vi "Initialize RT Driver.vi"(8 "error in":errorcluster, 10 "settings in":T18 {"objectData"."out object status BD"."Data Reference" format="%.0x"; "objectData"."out object data BD"."Data Reference" format="%.0x"; "objectData"."out interaction status BD"."Data Reference" format="%.0x"; "objectData"."out interaction data BD"."Data Reference" format="%.0x"}, 11 "Device Reference in":T25 format="%.0x") -> (0 "error out":errorcluster, 1 "inline runtime data":T1 {"out object status BD"."Data Reference" format="%.0x"; "out object data BD"."Data Reference" format="%.0x"; "out interaction status BD"."Data Reference" format="%.0x"; "out interaction data BD"."Data Reference" format="%.0x"}, 2 "settings out":T18 {"objectData"."out object status BD"."Data Reference" format="%.0x"; "objectData"."out object data BD"."Data Reference" format="%.0x"; "objectData"."out interaction status BD"."Data Reference" format="%.0x"; "objectData"."out interaction data BD"."Data Reference" format="%.0x"}, 3 "Device Reference out":T25 format="%.0x")   [LabVIEW 2019, in "HLA Custom Device Engine.lvlib"]
uses:
  HLA Custom Device Engine.lvlib
  <vilib>/NI VeriStand/Custom Device API/Custom Device Item Ref.ctl
  Shared/Compiled.Settings.ctl
  Shared/main_page_config.ctl
  Shared/object_managament_config.ctl
  Shared/interaction_parameter_configuration.ctl
  Shared/object_attribute_configuration.ctl
  Shared/object_status_info.ctl
  Shared/object_data.ctl
  <vilib>/NI VeriStand/Custom Device API/Block Data Reference.ctl
  <vilib>/NI VeriStand/Custom Device API/Data Reference.ctl
  RTruntimeData.ctl
  _typedefs/RThlaMapHelpers.ctl
  _typedefs/map_in_interaction.ctl
  _typedefs/map_interaction_value.ctl
  _typedefs/map_attr_param_data.ctl
  _typedefs/map_object.ctl
  _typedefs/map_object_key.ctl
  _typedefs/map_object_value.ctl
  _typedefs/map_object_instance.ctl
  _typedefs/map_object_instance_value.ctl
  _typedefs/map_object_vs_instance.ctl
  _typedefs/map_out_vs_ch_instanceId.ctl
  _typedefs/map_out_vs_ch_objects.ctl
  _typedefs/map_out_vs_ch_objects_value.ctl
  _typedefs/map_out_vs_ch_interactIonClass.ctl
  <vilib>/addons/hla/receiveInteractionEvent_type.ctl
  <vilib>/addons/hla/OrderType.ctl
  <vilib>/addons/hla/TransportationType.ctl
  <vilib>/addons/hla/reflectAttributeValuesEvent_type.ctl
  <vilib>/addons/hla/discoverObjectInstanceEvent_type.ctl
  <vilib>/addons/hla/removeObjectInstanceEvent_type.ctl
  Shared/rt_init_state.ctl
  <vilib>/Utility/miscctls.llb/LVMapReplaceAction.ctl
  _typedefs/discoverObjectInstance_type.ctl
  <vilib>/NI VeriStand/Custom Device API/Custom Device API.lvlib
  <vilib>/addons/hla/openrti_rti1516eLv.lvlib
  Shared/HLA Custom Device Shared.lvlib
  _Debug/VsDebugLibrary.lvlib
  <vilib>/addons/hla/helpers/ahs.lvlib
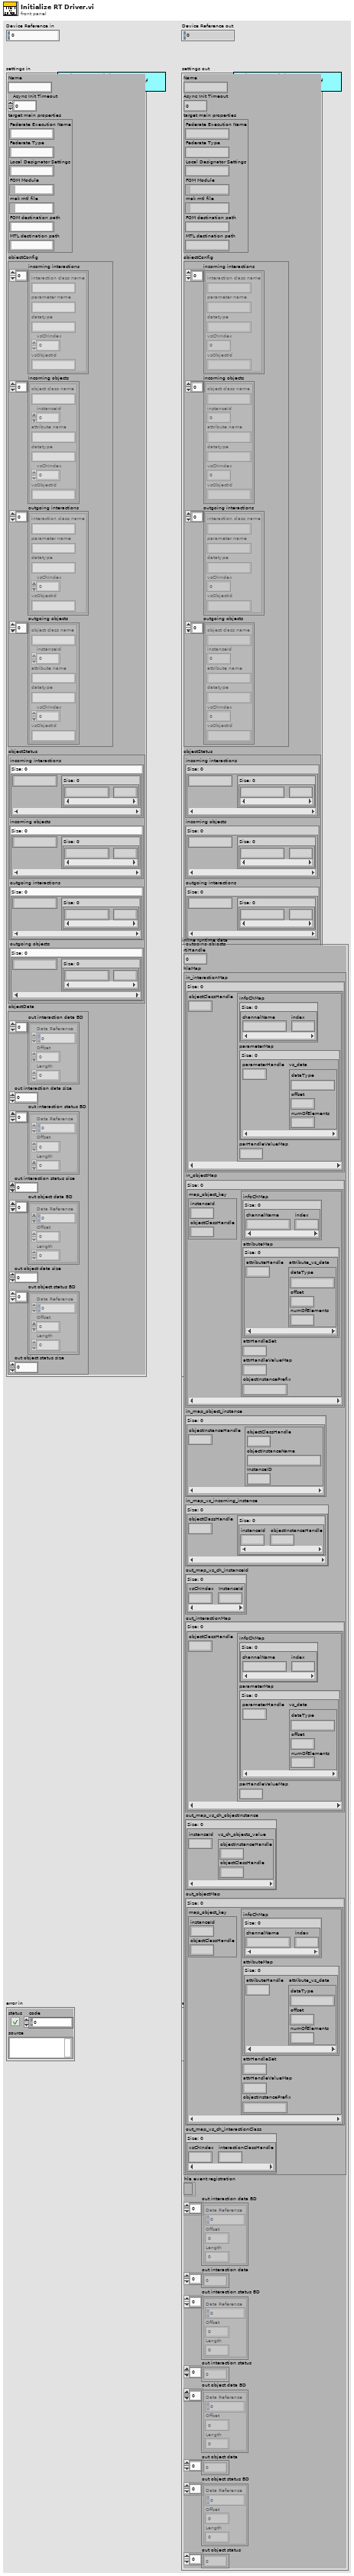
[diagram p1: front panel]
types:
  T1 = typedef "HLA Custom Device Engine.lvlib/RTruntimeData.ctl" = cluster{"rtiHandle":i64, "hlaMap":T2, "hla event registration":refnum<event-registration>, "out interaction data BD":T16[], "out interaction data":dbl[], "out interaction status BD":T16[], "out interaction status ":dbl[], "out object data BD":T16[], "out object data":dbl[], "out object status BD":T16[], "out object status ":dbl[]}
  T2 = typedef "HLA Custom Device Engine.lvlib/RThlaMapHelpers.ctl" = cluster{"in_interactionMap":T3, "in_objectMap":T6, "in_map_object_instance":T9, "in_map_vs_incoming_instance":T11, "out_map_vs_ch_instanceId":T12, "out_interactionMap":T3, "out_map_vs_ch_objectInstance":T13, "out_objectMap":T6, "out_map_vs_ch_interactionClass":T15}
  T3 = typedef "HLA Custom Device Engine.lvlib/map_in_interaction.ctl" = map{u64, T4}
  T4 = typedef "HLA Custom Device Engine.lvlib/map_interaction_value.ctl" = cluster{"infoChMap":map{string, i32}, "parameterMap":map{u64, T5}, "parHandleValueMap":u64}
  T5 = typedef "HLA Custom Device Engine.lvlib/map_attr_param_data.ctl" = cluster{"dataType":string, "offset":i32, "numOfElements":i32}
  T6 = typedef "HLA Custom Device Engine.lvlib/map_object.ctl" = map{T7, T8}
  T7 = typedef "HLA Custom Device Engine.lvlib/map_object_key.ctl" = cluster{"instanceId":i32, "objectClassHandle":u64}
  T8 = typedef "HLA Custom Device Engine.lvlib/map_object_value.ctl" = cluster{"infoChMap":map{string, i32}, "attributeMap":map{u64, T5}, "attrHandleSet":u64, "attrHandleValueMap":u64, "objectInstancePrefix":string}
  T9 = typedef "HLA Custom Device Engine.lvlib/map_object_instance.ctl" = map{u64, T10}
  T10 = typedef "HLA Custom Device Engine.lvlib/map_object_instance_value.ctl" = cluster{"objectClassHandle":u64, "objectInstanceName":string, "InstanceID":i32}
  T11 = typedef "HLA Custom Device Engine.lvlib/map_object_vs_instance.ctl" = map{u64, map{i32, u64}}
  T12 = typedef "HLA Custom Device Engine.lvlib/map_out_vs_ch_instanceId.ctl" = map{i32, i32}
  T13 = typedef "HLA Custom Device Engine.lvlib/map_out_vs_ch_objects.ctl" = map{i32, T14}
  T14 = typedef "HLA Custom Device Engine.lvlib/map_out_vs_ch_objects_value.ctl" = cluster{"objectInstanceHandle":u64, "objectClassHandle":u64}
  T15 = typedef "HLA Custom Device Engine.lvlib/map_out_vs_ch_interactIonClass.ctl" = map{i32, u64}
  T16 = typedef "Custom Device API.lvlib/Block Data Reference.ctl" = cluster{"Data Reference":T17, "Offset":u64, "Length":u64}
  T17 = typedef "Custom Device API.lvlib/Data Reference.ctl" = i32
  T18 = typedef "HLA Custom Device Shared.lvlib/Compiled.Settings.ctl" = cluster{"Name":string, "Async Init Timeout":u16, "target main properties":T19, "obiectConfig":T20, "objectStatus":T23, "objectData":T24}
  T19 = typedef "HLA Custom Device Shared.lvlib/main_page_config.ctl" = cluster{"Federate Execution Name":string, "Federate Type":string, "Local Designator Settings":string, "FOM Module":path, "mak mtl file":path, "FOM destination path":string, "MTL destination path":string}
  T20 = typedef "HLA Custom Device Shared.lvlib/object_managament_config.ctl" = cluster{"incoming interactions":T21[], "incoming objects":T22[], "outgoing interactions":T21[], "outgoing objects":T22[]}
  T21 = typedef "HLA Custom Device Shared.lvlib/interaction_parameter_configuration.ctl" = cluster{"interaction class name":string, "parameter name":string, "datatype":string, "vsChIndex":i32, "vsObjectId":string}
  T22 = typedef "HLA Custom Device Shared.lvlib/object_attribute_configuration.ctl" = cluster{"object class name":string, "instanceId":i32, "attribute name":string, "datatype":string, "vsChIndex":i32, "vsObjectId":string}
  T23 = typedef "HLA Custom Device Shared.lvlib/object_status_info.ctl" = cluster{"incoming interactions":map{string, map{string, i32}}, "incoming objects":map{string, map{string, i32}}, "outgoing interactions":map{string, map{string, i32}}, "outgoing objects":map{string, map{string, i32}}}
  T24 = typedef "HLA Custom Device Shared.lvlib/object_data.ctl" = cluster{"out interaction data BD":T16[], "out interaction data size":i32, "out interaction status BD":T16[], "out interaction status size":i32, "out object data BD":T16[], "out object data size":i32, "out object status BD":T16[], "out object status size":i32}
  T25 = typedef "Custom Device API.lvlib/Custom Device Item Ref.ctl" = u64
  T26 = typedef "HLA Custom Device Shared.lvlib/rt_init_state.ctl" = enum16{"Initialize", "Connect", "FOM Management", "Object Management", "Start", "RegisterObjectInstances"}
  T27 = cluster{"objInstanceName":string, "success":bool}
  T28 = typedef "LVMapReplaceAction.ctl" = enum32{"Modify Entry only if found", "Add or Modify Entry", "Delete Entry"}
  T29 = typedef "HLA Custom Device Engine.lvlib/discoverObjectInstance_type.ctl" = cluster{"objectInstanceHandle":u64, "objectClassHandle":u64, "objectInstanceName":string}
  T30 = cluster{"[0]":u8, "[1]":u8, "[2]":u8, "[3]":u8, "[4]":u8, "[5]":u8, "[6]":u8, "[7]":u8, "[8]":u8, "[9]":u8, "[10]":u8, "[11]":u8, "[12]":u8, "[13]":u8, "[14]":u8, "[15]":u8, "[16]":u8, "[17]":u8, "[18]":u8, "[19]":u8, "[20]":u8, "[21]":u8, "[22]":u8, "[23]":u8, "[24]":u8, "[25]":u8, "[26]":u8, "[27]":u8, "[28]":u8, "[29]":u8, "[30]":u8, "[31]":u8, "[32]":u8, "[33]":u8, "[34]":u8, "[35]":u8, "[36]":u8, "[37]":u8, "[38]":u8, "[39]":u8, "[40]":u8, "[41]":u8, "[42]":u8, "[43]":u8, "[44]":u8, "[45]":u8, "[46]":u8, "[47]":u8, "[48]":u8, "[49]":u8, "[50]":u8, "[51]":u8, "[52]":u8, "[53]":u8, "[54]":u8, "[55]":u8, "[56]":u8, "[57]":u8, "[58]":u8, "[59]":u8, "[60]":u8, "[61]":u8, "[62]":u8, "[63]":u8, "[64]":u8, "[65]":u8, "[66]":u8, "[67]":u8, "[68]":u8, "[69]":u8, "[70]":u8, "[71]":u8, "[72]":u8, "[73]":u8, "[74]":u8, "[75]":u8, "[76]":u8, "[77]":u8, "[78]":u8, "[79]":u8, "[80]":u8, "[81]":u8, "[82]":u8, "[83]":u8, "[84]":u8, "[85]":u8, "[86]":u8, "[87]":u8, "[88]":u8, "[89]":u8, "[90]":u8, "[91]":u8, "[92]":u8, "[93]":u8, "[94]":u8, "[95]":u8, "[96]":u8, "[97]":u8, "[98]":u8, "[99]":u8, "[100]":u8, "[101]":u8, "[102]":u8, "[103]":u8, "[104]":u8, "[105]":u8, "[106]":u8, "[107]":u8, "[108]":u8, "[109]":u8, "[110]":u8, "[111]":u8, "[112]":u8, "[113]":u8, "[114]":u8, "[115]":u8, "[116]":u8, "[117]":u8, "[118]":u8, "[119]":u8, "[120]":u8, "[121]":u8, "[122]":u8, "[123]":u8, "[124]":u8, "[125]":u8, "[126]":u8, "[127]":u8}
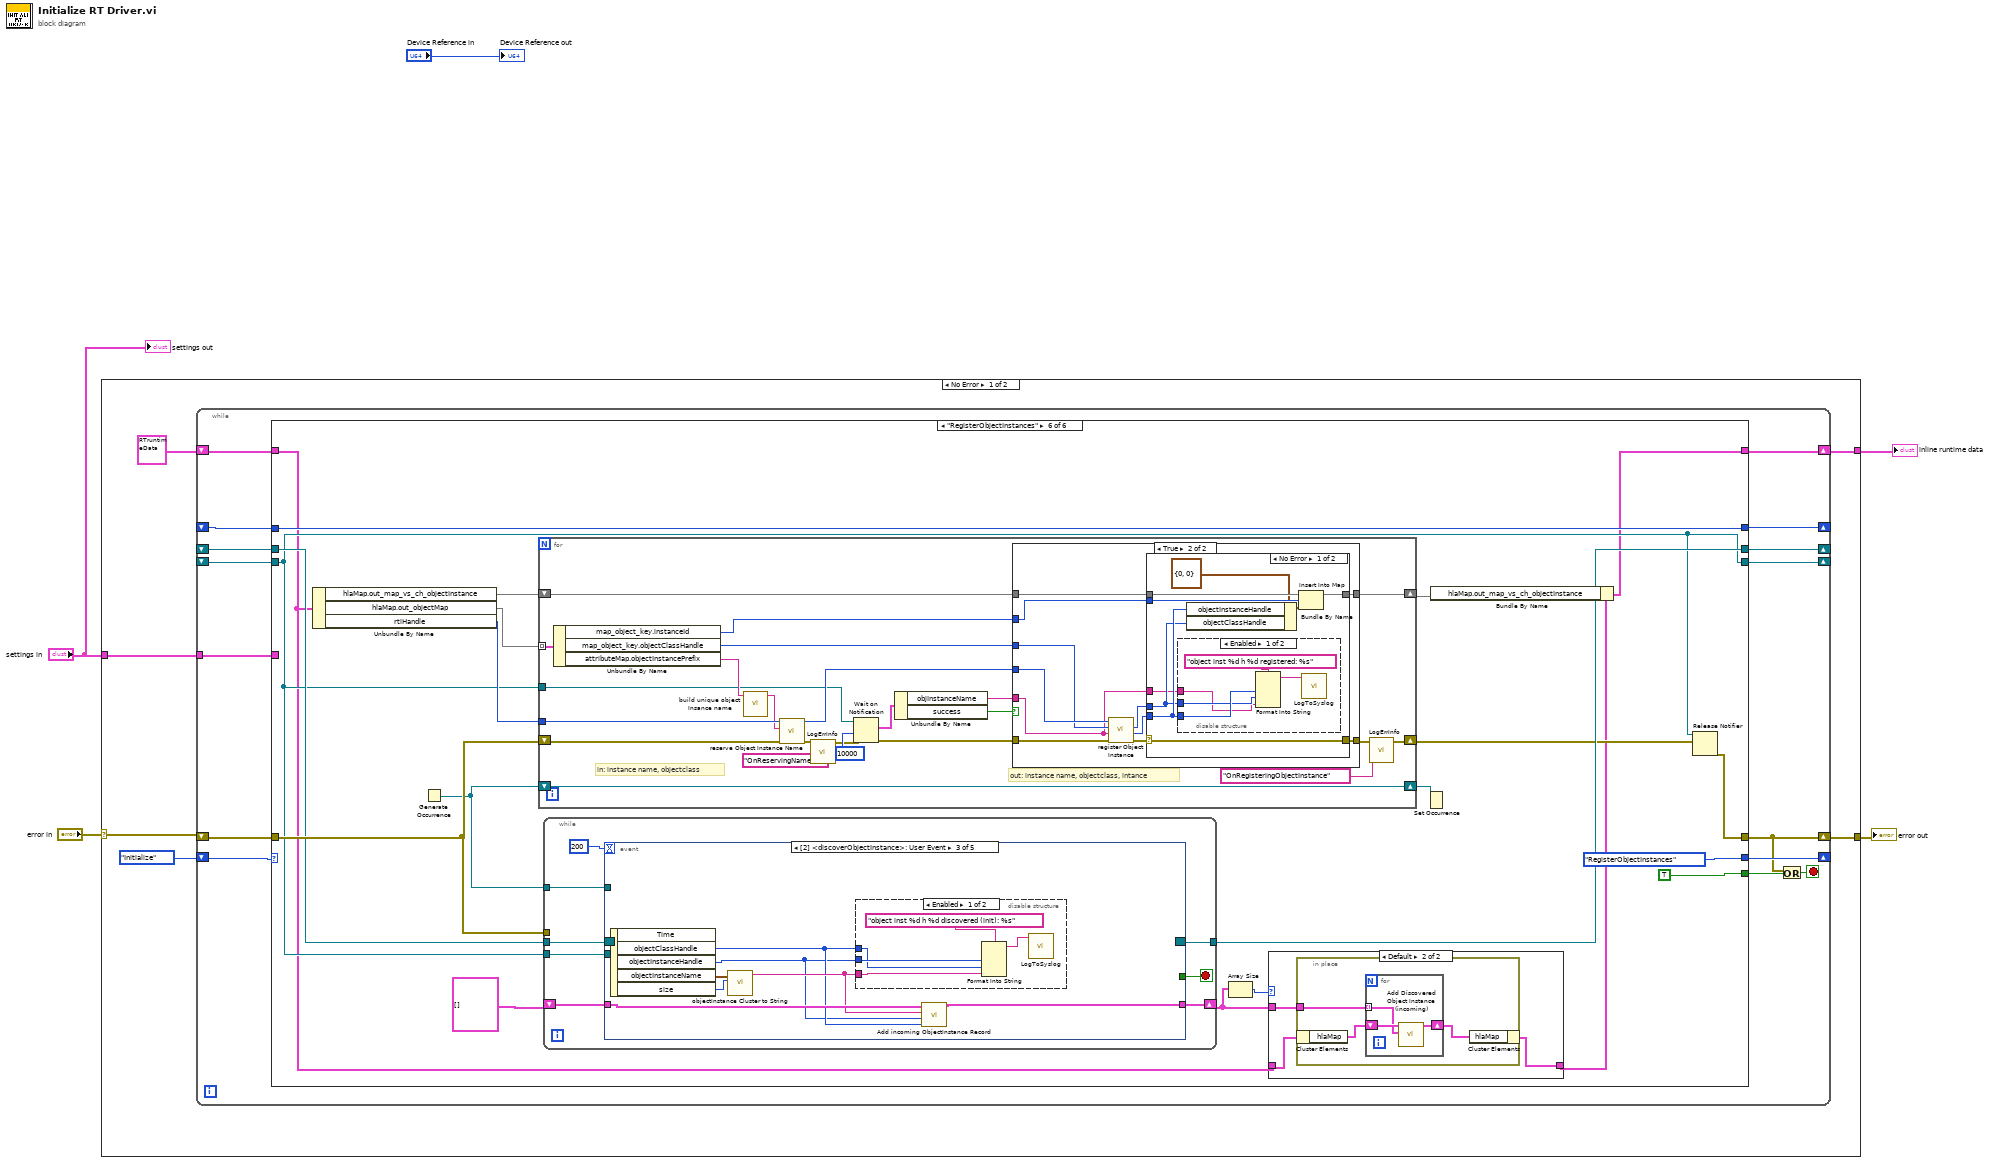
[diagram p0: block diagram]
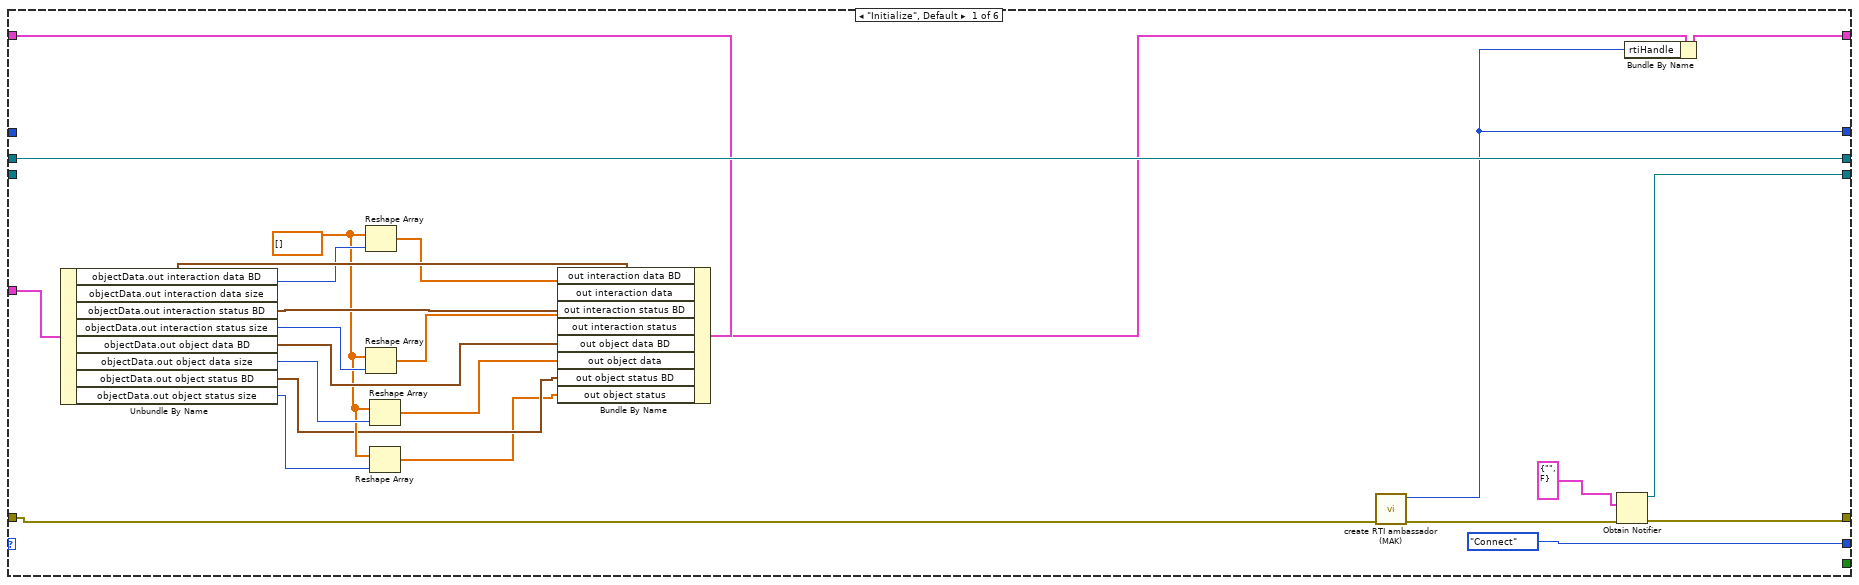
[diagram p2: hidden frame]
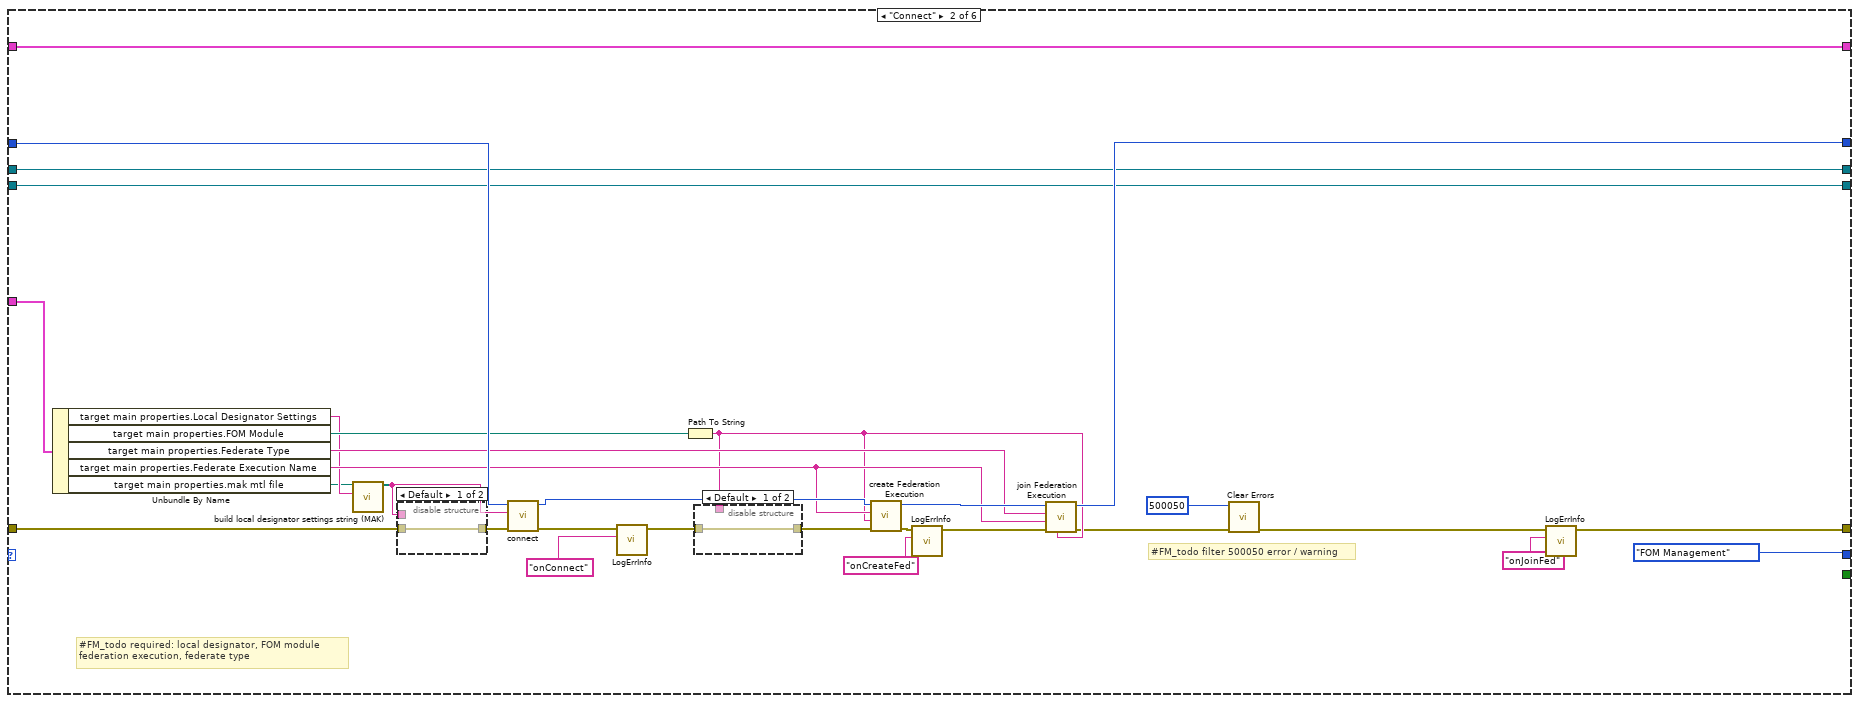
[diagram p3: hidden frame]
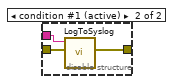
[diagram p4: hidden frame]
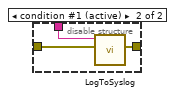
[diagram p5: hidden frame]
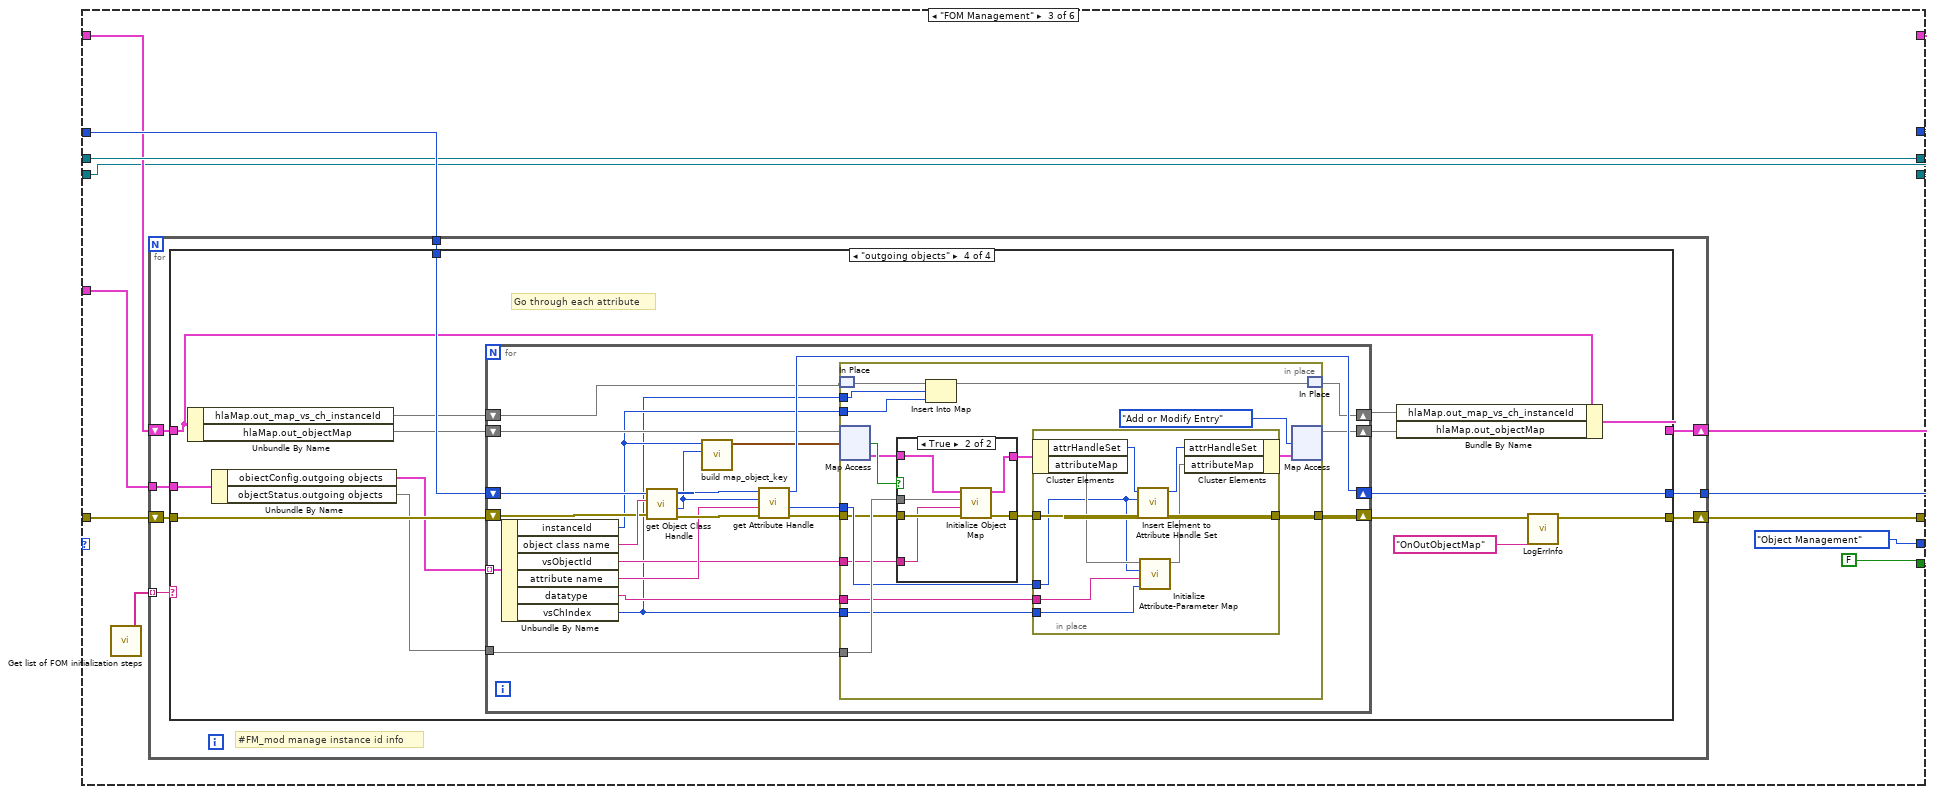
[diagram p6: hidden frame]
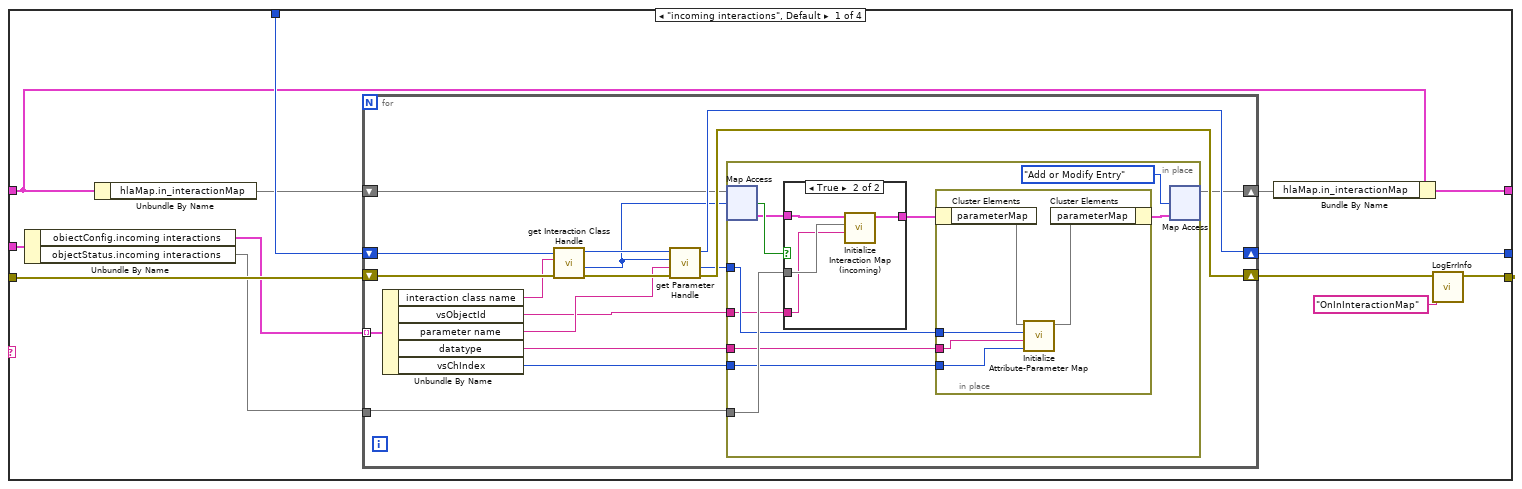
[diagram p7: hidden frame]
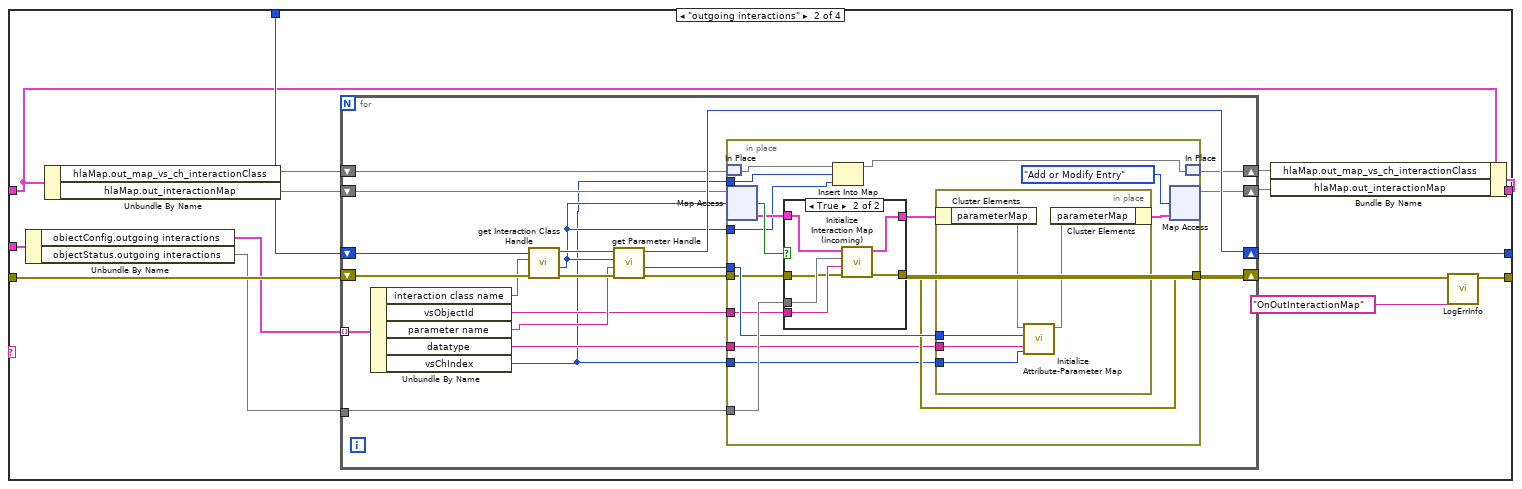
[diagram p9: hidden frame]
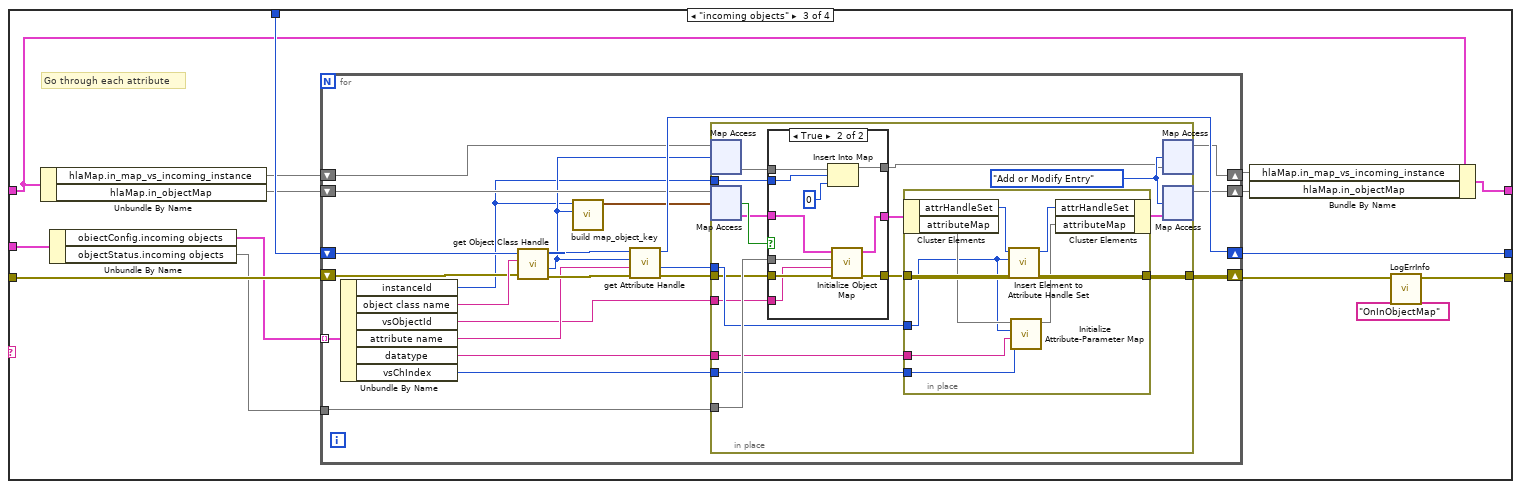
[diagram p11: hidden frame]
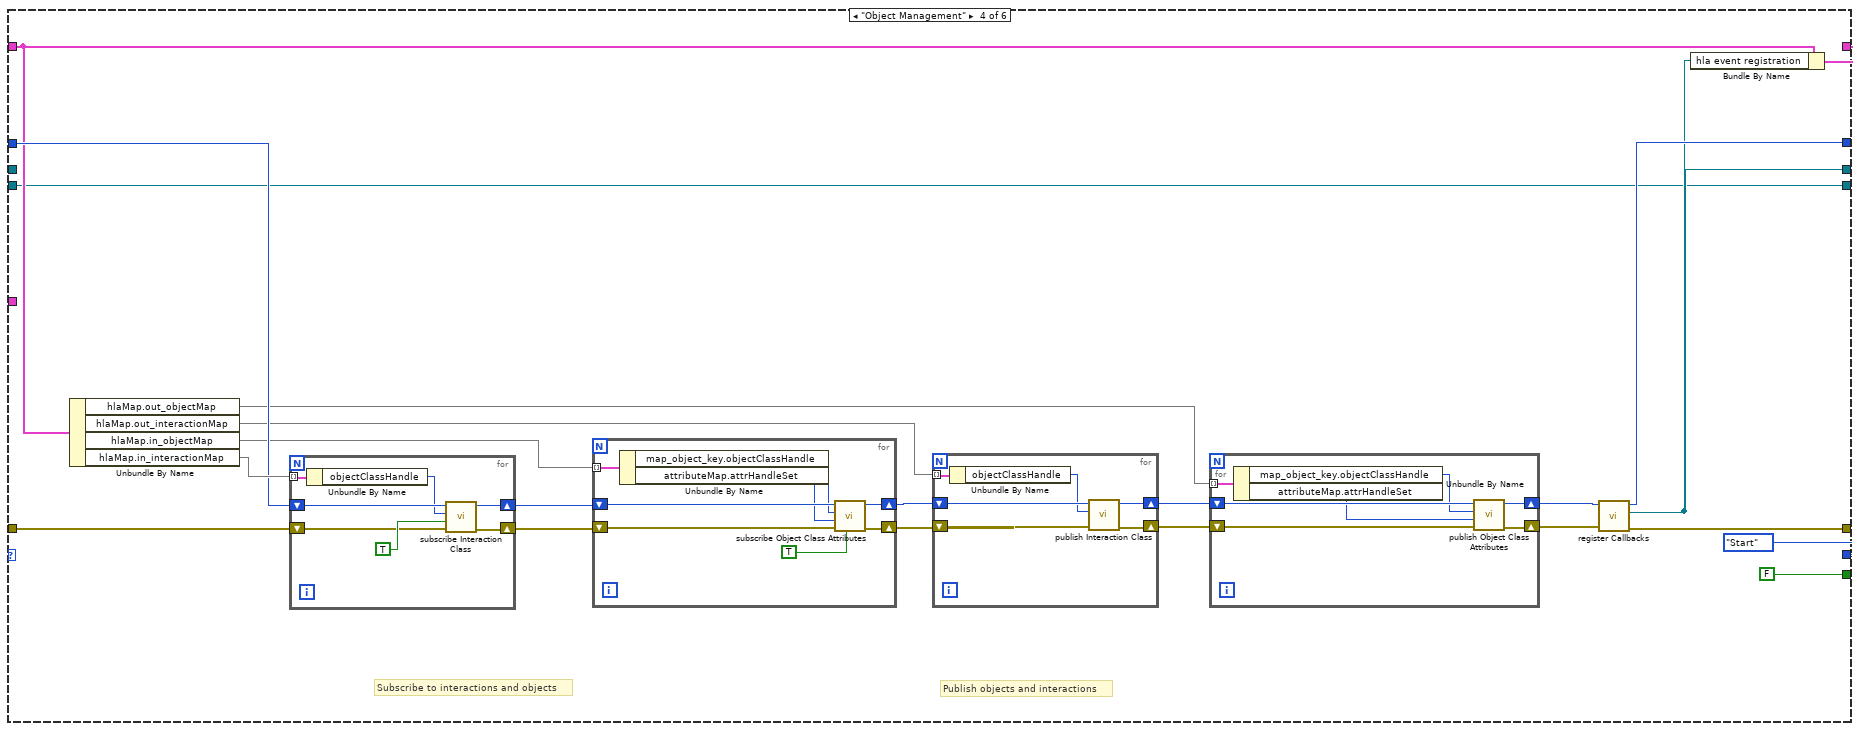
[diagram p14: hidden frame]
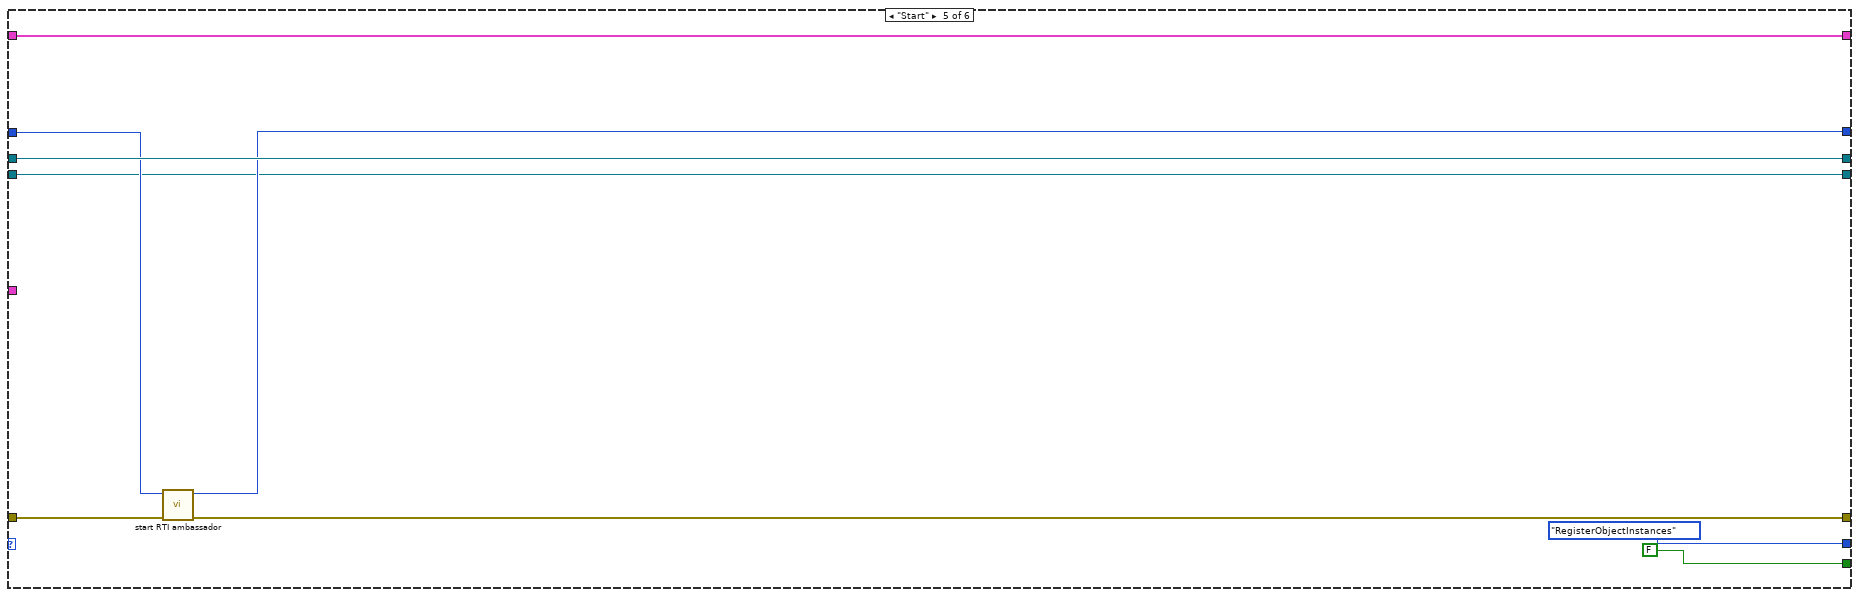
[diagram p15: hidden frame]
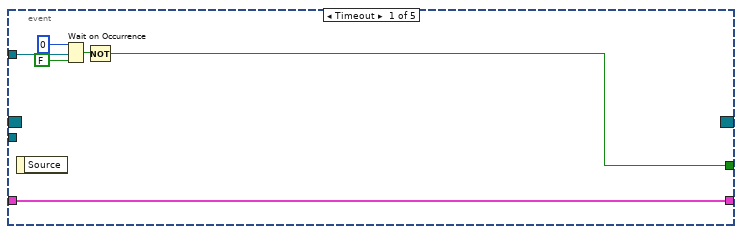
[diagram p20: hidden frame]
diagram:
  n1 = case shown="No Error" "error in" {
    selector: "error in" -> [w10 w559]
    tunnel: "settings in" -> [w9 _]
    tunnel: [w8 w559] -> w2
    tunnel: [w6 _] -> w1
    frame No Error {
      n2 = while {
        shift-right: [w25] -> _
        shift-left: rt_init_state."Initialize" -> [w26]
        tunnel: w9 -> [w24]
        shift-right: [w19] -> w8
        shift-left: w10 -> [w23]
        shift-right: [w22] -> _
        shift-left: _ -> [w21]
        shift-right: [w17] -> _
        shift-left: _ -> [w16]
        shift-right: [w14] -> w6
        shift-left: T1 {"rtiHandle"=0, "hlaMap"={"in_interactionMap"={}, "in_objectMap"={}, "in_map_object_instance"={}, "in_map_vs_incoming_instance"={}, "out_map_vs_ch_instanceId"={}, "out_interactionMap"={}, "out_map_vs_ch_objectInstance"={}, "out_objectMap"={}, "out_map_vs_ch_interactionClass"={}}, "hla event registration"=refnum, "out interaction data BD"=[], "out interaction data"=[], "out interaction status BD"=[], "out interaction status "=[], "out object data BD"=[], "out object data"=[], "out object status BD"=[], "out object status "=[]} ("inline runtime data") -> [w15]
        shift-right: [w13] -> _
        shift-left: _ -> [w12]
        stop <- w18 stop-if-true
        n3 = case shown="\"RegisterObjectInstances\"" w26 {
          tunnel: [w36 w72 w96 w383 w423 w440] -> w19
          tunnel: [_ _ FALSE FALSE FALSE TRUE] -> w20
          tunnel: [rt_init_state."Connect" rt_init_state."FOM Management" rt_init_state."Object Management" rt_init_state."Start" rt_init_state."RegisterObjectInstances" rt_init_state."RegisterObjectInstances"] -> w25
          tunnel: w24 -> [w48 w56 w94 _ _ _]
          tunnel: w23 -> [w50 w63 w99 w389 w427 w445]
          tunnel: [w42 w75 w97 w386 w425 w449] -> w22
          tunnel: w21 -> [_ w80 w98 w387 w426 w449]
          tunnel: [w49 w55 w93 w380 w428 w446] -> w17
          tunnel: w16 -> [w49 w55 w93 _ w428 w443]
          tunnel: w15 -> [w47 w54 w92 w379 w421 w432]
          tunnel: [w43 w54 w91 w381 w421 w437] -> w14
          tunnel: [w35 w53 w90 w375 w420 w439] -> w13
          tunnel: w12 -> [_ w53 w90 w375 w420 w439]
          frame "Initialize", Default {
            w31 = dbl[] [] ("out interaction data")
            n4 = Unbundle By Name(w48) -> ("objectData.out interaction data BD"=w46:T16[], "objectData.out interaction data size"=w41:i32, "objectData.out interaction status BD"=w45:T16[], "objectData.out interaction status size"=w39:i32, "objectData.out object data BD"=w33:T16[], "objectData.out object data size"=w32:i32, "objectData.out object status BD"=w29:T16[], "objectData.out object status size"=w28:i32)
            n5 = Reshape Array(w31, w41) -> (w40:dbl[])
            n6 = Reshape Array(w31, w39) -> (w38:dbl[])
            n7 = Reshape Array(w31, w32) -> (w30:dbl[])
            n8 = Reshape Array(w31, w28) -> (w27:dbl[])
            n9 = Bundle By Name(cluster=w47, "out interaction data BD"=w46, "out interaction data"=w40, "out interaction status BD"=w45, "out interaction status"=w38, "out object data BD"=w33, "out object data"=w30, "out object status BD"=w29, "out object status"=w27) -> (w44:T1)
            n10 = call <vilib>:"create RTI ambassador (MAK).vi"("error in"=w50) -> ("error out"=w37:errorcluster, "rtiHandle out"=w42:i64)  [unwired: 9 in]
            n11 = Obtain Notifier(notification data type=T27 {"objInstanceName"="", "success"=FALSE} ("notification"), error in (no error)=w37) -> (notifier out=w35:refnum<notifier>, error out=w36:errorcluster)  [unwired: 2 in, 1 out]
            n12 = Bundle By Name(cluster=w44, "rtiHandle"=w42) -> (w43:T1)
          }
          frame "Connect" {
            # "#FM_todo filter 500050 error / warning"
            # "#FM_todo required: local designator, FOM module\nfederation execution, federate type"
            n13 = Unbundle By Name(w56) -> ("target main properties.Local Designator Settings"=w66:string, "target main properties.FOM Module"=w69:path, "target main properties.Federate Type"=w68:string, "target main properties.Federate Execution Name"=w67:string, "target main properties.mak mtl file"=w65:path)
            n14 = call "build local designator settings string (MAK).vi"("configuration string"=w66, "configuration file"=w65) -> ("local designator settings"=w64:string)  [unwired: 9 in]
            n15 = disable-structure shown="Default" {
              disable-tunnel: w64 -> [_ w85]
              disable-tunnel: w63 -> [w82 w84]
              disable-tunnel: [w82 w83] -> w62
              frame condition #0 {
              }
              frame condition #1 (active) {
                n16 = call "LogToSyslog.vi"("error in (no error)"=w84, "message"=w85) -> ("error out"=w83:errorcluster)  [unwired: 8 in, 1 out]
              }
            }
            n17 = call <vilib>:"connect.vi"("error in"=w62, "rtinode address"=w64, "rtiHandle in"=w80) -> ("error out"=w77:errorcluster, "rtiHandle out"=w76:i64)  [unwired: 7 in]
            n18 = call "LogErrInfo.vi"("location info"="onConnect", "error in (no error)"=w77) -> ("error out"=w61:errorcluster)  [unwired: 9 in]
            n19 = Path To String(path=w69) -> (string=w59:string)
            n20 = disable-structure shown="Default" {
              disable-tunnel: w61 -> [w86 w89]
              disable-tunnel: [w86 w88] -> w60
              disable-tunnel: w59 -> [_ w87]
              frame condition #0 {
              }
              frame condition #1 (active) {
                n21 = call "LogToSyslog.vi"("error in (no error)"=w89, "message"=w87) -> ("error out"=w88:errorcluster)  [unwired: 8 in, 1 out]
              }
            }
            n22 = call <vilib>:"create Federation Execution.vi"("error in"=w60, "fomModules"=w59, "federationExecutionName"=w67, "rtiHandle in"=w76) -> ("error out"=w78:errorcluster, "rtiHandle out"=w79:i64)  [unwired: 6 in]
            n23 = call "LogErrInfo.vi"("location info"="onCreateFed", "error in (no error)"=w78) -> ("error out"=w73:errorcluster)  [unwired: 9 in]
            n24 = call <vilib>:"join Federation Execution.vi"("additionalFomModules(\"\")"=w59, "error in"=w73, "federationExecutionName"=w67, "federateType"=w68, "rtiHandle in"=w79) -> ("error out"=w58:errorcluster, "rtiHandle out"=w75:i64)  [unwired: 5 in]
            n25 = call <vilib>:"Clear Errors.vi"("error in (no error)"=w58, "specific error code to clear (0: all)"=500050) -> ("error out"=w57:errorcluster)  [unwired: 4 in, 1 out]
            n26 = call "LogErrInfo.vi"("location info"="onJoinFed", "error in (no error)"=w57) -> ("error out"=w72:errorcluster)  [unwired: 9 in]
          }
          frame "FOM Management" {
            n27 = call "Get list of FOM initialization steps.vi"() -> ("init steps"=w95:string[])  [unwired: 11 in]
            n28 = for {
              tunnel: w94 -> [w109]
              tunnel: w98 -> [w107]
              tunnel: [w105] -> w97
              shift-right: [w103] -> w96
              shift-left: w99 -> [w108]
              shift-right: [w104] -> w91
              shift-left: w92 -> [w106]
              tunnel: w95 -> [w102] mode=indexing
              # "#FM_mod manage instance id info"
              n29 = case shown="\"outgoing objects\"" w102 {
                tunnel: w109 -> [w122 w174 w238 w313]
                tunnel: w108 -> [w121 w173 w237 w312]
                tunnel: w107 -> [w119 w171 w235 w310]
                tunnel: w106 -> [w117 w169 w233 w308]
                tunnel: [w116 w168 w232 w307] -> w105
                tunnel: [w115 w167 w231 w306] -> w104
                tunnel: [w112 w165 w228 w303] -> w103
                frame "incoming interactions", Default {
                  n30 = Unbundle By Name(w122) -> ("obiectConfig.incoming interactions"=w120:T21[], "objectStatus.incoming interactions"=w110:map{string, map{string, i32}})
                  n31 = Unbundle By Name(w117) -> ("hlaMap.in_interactionMap"=w118:T3)
                  n32 = for {
                    tunnel: w120 -> [w139] mode=indexing
                    shift-right: [w133] -> w116
                    shift-left: w119 -> [w137]
                    shift-right: [w132] -> w113
                    shift-left: w121 -> [w136]
                    shift-right: [w128] -> w114
                    shift-left: w118 -> [w131]
                    tunnel: w110 -> [w129]
                    n33 = Unbundle By Name(w139) -> ("interaction class name"=w126:string, "vsObjectId"=w125:string, "parameter name"=w134:string, "datatype"=w124:string, "vsChIndex"=w123:i32)
                    n34 = call <vilib>:"get Interaction Class Handle.vi"("error in"=w136, "interaction class name"=w126, "rtiHandle in"=w137) -> ("error out"=w138:errorcluster, "intClassHandle"=w130:u64, "rtiHandle out"=w135:i64)  [unwired: 6 in]
                    n35 = call <vilib>:"get Parameter Handle.vi"("error in"=w138, "theName"=w134, "intClassHandle"=w130, "rtiHandle in"=w135) -> ("error out"=w132:errorcluster, "parameterHandle"=w127:u64, "rtiHandle out"=w133:i64)  [unwired: 5 in]
                    n36 = in-place {
                      in-place-border: w129 -> [w148]
                      in-place-border: w127 -> [w144]
                      in-place-border: w125 -> [w142]
                      in-place-border: w124 -> [w141]
                      in-place-border: w123 -> [w140]
                      n37 = in-place-map #1(w131, w130) -> (w147:T4, w149:bool)  [unwired: 1 in]
                      n38 = case shown="True" w149 {
                        tunnel: w148 -> [_ w159]
                        tunnel: w147 -> [w155 w158]
                        tunnel: [w155 w157] -> w145
                        tunnel: w142 -> [_ w156]
                        frame False {
                        }
                        frame True {
                          n39 = call "Initialize Interaction Map (incoming).vi"("vsObjectId"=w156, "incoming interactions"=w159, "in_interaction map in"=w158) -> ("in_interaction map out"=w157:T4)  [unwired: 7 in, 1 out]
                        }
                      }
                      n40 = in-place {
                        in-place-border: w144 -> [w153]
                        in-place-border: w141 -> [w151]
                        in-place-border: w140 -> [w150]
                        n41 = in-place-cluster #2(w145) -> ("parameterMap"=w154:map{u64, T5})
                        n42 = call "Initialize Attribute-Parameter Map.vi"("vs channel index"=w150, "dataType"=w151, "parameterHandle"=w153, "Map in"=w154) -> ("Map out"=w152:map{u64, T5})  [unwired: 7 in]
                        n43 = in-place-cluster #2("parameterMap"=w152) -> (w143:T4)
                      }
                      n44 = in-place-map #1(w143, LVMapReplaceAction."Add or Modify Entry" ("action")) -> (w128:T3)  [unwired: 2 out]
                    }
                  }
                  n45 = Bundle By Name(cluster=w117, "hlaMap.in_interactionMap"=w114) -> (w115:T1)
                  n46 = call "LogErrInfo.vi"("location info"="OnInInteractionMap", "error in (no error)"=w113) -> ("error out"=w112:errorcluster)  [unwired: 9 in]
                }
                frame "outgoing interactions" {
                  n47 = Unbundle By Name(w174) -> ("obiectConfig.outgoing interactions"=w172:T21[], "objectStatus.outgoing interactions"=w163:map{string, map{string, i32}})
                  n48 = Unbundle By Name(w169) -> ("hlaMap.out_map_vs_ch_interactionClass"=w162:T15, "hlaMap.out_interactionMap"=w170:T3)
                  n49 = for {
                    tunnel: w172 -> [w194] mode=indexing
                    shift-right: [w188] -> w168
                    shift-left: w171 -> [w192]
                    shift-right: [w177] -> w166
                    shift-left: w173 -> [w191]
                    shift-right: [w185] -> w161
                    shift-left: w170 -> [w187]
                    tunnel: w163 -> [w186]
                    shift-right: [w179] -> w160
                    shift-left: w162 -> [w181]
                    n50 = Unbundle By Name(w194) -> ("interaction class name"=w183:string, "vsObjectId"=w182:string, "parameter name"=w189:string, "datatype"=w176:string, "vsChIndex"=w175:i32)
                    n51 = call <vilib>:"get Interaction Class Handle.vi"("error in"=w191, "interaction class name"=w183, "rtiHandle in"=w192) -> ("error out"=w193:errorcluster, "intClassHandle"=w180:u64, "rtiHandle out"=w190:i64)  [unwired: 6 in]
                    n52 = call <vilib>:"get Parameter Handle.vi"("error in"=w193, "theName"=w189, "intClassHandle"=w180, "rtiHandle in"=w190) -> ("error out"=w178:errorcluster, "parameterHandle"=w184:u64, "rtiHandle out"=w188:i64)  [unwired: 5 in]
                    n53 = in-place {
                      in-place-border: w186 -> [w209]
                      in-place-border: w184 -> [w205]
                      in-place-border: w182 -> [w203]
                      in-place-border: w175 -> [w198]
                      in-place-border: w180 -> [w197]
                      in-place-border: w178 -> [w202]
                      in-place-border: [w201] -> w177
                      in-place-border: w176 -> [w196]
                      in-place-border: w175 -> [w195]
                      n54 = in-place-match #3(w181) -> (w200:T15)
                      n55 = in-place-map #4(w187, w180) -> (w208:T4, w210:bool)  [unwired: 1 in]
                      n56 = case shown="True" w210 {
                        tunnel: w209 -> [_ w223]
                        tunnel: w208 -> [w217 w222]
                        tunnel: [w217 w221] -> w206
                        tunnel: w203 -> [_ w220]
                        tunnel: w202 -> [w216 w219]
                        tunnel: [w216 w218] -> w201
                        frame False {
                        }
                        frame True {
                          n57 = call "Initialize Interaction Map (incoming).vi"("error in"=w219, "vsObjectId"=w220, "incoming interactions"=w223, "in_interaction map in"=w222) -> ("error out"=w218:errorcluster, "in_interaction map out"=w221:T4)  [unwired: 6 in]
                        }
                      }
                      n58 = Insert Into Map(map in=w200, key=w198, value=w197) -> (map out=w199:T15)  [unwired: 2 out]
                      n59 = in-place {
                        in-place-border: w205 -> [w213]
                        in-place-border: w196 -> [w212]
                        in-place-border: w195 -> [w211]
                        n60 = in-place-cluster #5(w206) -> ("parameterMap"=w215:map{u64, T5})
                        n61 = call "Initialize Attribute-Parameter Map.vi"("vs channel index"=w211, "dataType"=w212, "parameterHandle"=w213, "Map in"=w215) -> ("Map out"=w214:map{u64, T5})  [unwired: 7 in]
                        n62 = in-place-cluster #5("parameterMap"=w214) -> (w204:T4)
                      }
                      n63 = in-place-map #4(w204, LVMapReplaceAction."Add or Modify Entry" ("action")) -> (w185:T3)  [unwired: 2 out]
                      n64 = in-place-match #3(w199) -> (w179:T15)
                    }
                  }
                  n65 = Bundle By Name(cluster=w169, "hlaMap.out_map_vs_ch_interactionClass"=w160, "hlaMap.out_interactionMap"=w161) -> (w167:T1)
                  n66 = call "LogErrInfo.vi"("location info"="OnOutInteractionMap", "error in (no error)"=w166) -> ("error out"=w165:errorcluster)  [unwired: 9 in]
                }
                frame "incoming objects" {
                  # "Go through each attribute"
                  n67 = Unbundle By Name(w233) -> ("hlaMap.in_map_vs_incoming_instance"=w225:T11, "hlaMap.in_objectMap"=w234:T6)
                  n68 = Unbundle By Name(w238) -> ("obiectConfig.incoming objects"=w236:T22[], "objectStatus.incoming objects"=w226:map{string, map{string, i32}})
                  n69 = for {
                    tunnel: w236 -> [w260] mode=indexing
                    shift-right: [w255] -> w232
                    shift-left: w235 -> [w258]
                    shift-right: [w247] -> w229
                    shift-left: w237 -> [w249]
                    shift-right: [w252] -> w230
                    shift-left: w234 -> [w254]
                    tunnel: w226 -> [w253]
                    shift-right: [w243] -> w224
                    shift-left: w225 -> [w245]
                    n70 = Unbundle By Name(w260) -> ("instanceId"=w242:i32, "object class name"=w250:string, "vsObjectId"=w239:string, "attribute name"=w256:string, "datatype"=w241:string, "vsChIndex"=w240:i32)
                    n71 = call <vilib>:"get Object Class Handle.vi"("error in"=w249, "object name"=w250, "rtiHandle in"=w258) -> ("error out"=w259:errorcluster, "objectClassHandle"=w244:u64, "rtiHandle out"=w257:i64)  [unwired: 6 in]
                    n72 = call "build map_object_key.vi"("objectClassHandle"=w244, "instanceId"=w242) -> ("object_map_key"=w246:T7)  [unwired: 9 in]
                    n73 = call <vilib>:"get Attribute Handle.vi"("error in"=w259, "attribute name"=w256, "objectClassHandle in"=w244, "rtiHandle in"=w257) -> ("error out"=w248:errorcluster, "attributeHandle"=w251:u64, "rtiHandle out"=w255:i64)  [unwired: 4 in, 1 out]
                    n74 = in-place {
                      in-place-border: w253 -> [w275]
                      in-place-border: w251 -> [w272]
                      in-place-border: w248 -> [w270]
                      in-place-border: [w268] -> w247
                      in-place-border: w239 -> [w267]
                      in-place-border: w242 -> [w263]
                      in-place-border: w241 -> [w262]
                      in-place-border: w240 -> [w261]
                      w266 = LVMapReplaceAction."Add or Modify Entry" ("action")
                      n75 = in-place-map #6(w245, w244) -> (w265:map{i32, u64})  [unwired: 1 in, 1 out]
                      n76 = in-place-map #7(w254, w246) -> (w274:T8, w276:bool)  [unwired: 1 in]
                      n77 = case shown="True" w276 {
                        tunnel: w275 -> [_ w298]
                        tunnel: w274 -> [w288 w297]
                        tunnel: [w288 w296] -> w273
                        tunnel: w270 -> [w287 w295]
                        tunnel: [w287 w294] -> w269
                        tunnel: w267 -> [_ w293]
                        tunnel: w265 -> [w286 w292]
                        tunnel: [w286 w291] -> w264
                        tunnel: w263 -> [_ w290]
                        frame False {
                        }
                        frame True {
                          n78 = Insert Into Map(map in=w292, key=w290, value=u64 0) -> (map out=w291:map{i32, u64})  [unwired: 2 out]
                          n79 = call "Initialize Object Map.vi"("error in"=w295, "vsObjectId"=w293, "status channel map"=w298, "object map in"=w297) -> ("error out"=w294:errorcluster, "object map out"=w296:T8)  [unwired: 6 in]
                        }
                      }
                      n80 = in-place {
                        in-place-border: w272 -> [w281]
                        in-place-border: w269 -> [w285]
                        in-place-border: [w284] -> w268
                        in-place-border: w262 -> [w278]
                        in-place-border: w261 -> [w277]
                        n81 = in-place-cluster #8(w273) -> ("attrHandleSet"=w283:u64, "attributeMap"=w282:map{u64, T5})
                        n82 = call <vilib>:"Insert Element to Attribute Handle Set.vi"("error in"=w285, "attributeHandle"=w281, "attrHandleSet in"=w283) -> ("error out"=w284:errorcluster, "attrHandleSet out"=w279:u64)  [unwired: 6 in, 1 out]
                        n83 = call "Initialize Attribute-Parameter Map.vi"("vs channel index"=w277, "dataType"=w278, "parameterHandle"=w281, "Map in"=w282) -> ("Map out"=w280:map{u64, T5})  [unwired: 7 in]
                        n84 = in-place-cluster #8("attrHandleSet"=w279, "attributeMap"=w280) -> (w271:T8)
                      }
                      n85 = in-place-map #6(w264, w266) -> (w243:T11)  [unwired: 2 out]
                      n86 = in-place-map #7(w271, w266) -> (w252:T6)  [unwired: 2 out]
                    }
                  }
                  n87 = Bundle By Name(cluster=w233, "hlaMap.in_map_vs_incoming_instance"=w224, "hlaMap.in_objectMap"=w230) -> (w231:T1)
                  n88 = call "LogErrInfo.vi"("location info"="OnInObjectMap", "error in (no error)"=w229) -> ("error out"=w228:errorcluster)  [unwired: 9 in]
                }
                frame "outgoing objects" {
                  # "Go through each attribute"
                  n89 = Unbundle By Name(w308) -> ("hlaMap.out_map_vs_ch_instanceId"=w300:T12, "hlaMap.out_objectMap"=w309:T6)
                  n90 = Unbundle By Name(w313) -> ("obiectConfig.outgoing objects"=w311:T22[], "objectStatus.outgoing objects"=w301:map{string, map{string, i32}})
                  n91 = for {
                    tunnel: w311 -> [w335] mode=indexing
                    shift-right: [w330] -> w307
                    shift-left: w310 -> [w333]
                    shift-right: [w322] -> w304
                    shift-left: w312 -> [w324]
                    shift-right: [w327] -> w305
                    shift-left: w309 -> [w329]
                    tunnel: w301 -> [w328]
                    shift-right: [w316] -> w299
                    shift-left: w300 -> [w317]
                    n92 = Unbundle By Name(w335) -> ("instanceId"=w318:i32, "object class name"=w325:string, "vsObjectId"=w320:string, "attribute name"=w331:string, "datatype"=w315:string, "vsChIndex"=w314:i32)
                    n93 = call <vilib>:"get Object Class Handle.vi"("error in"=w324, "object name"=w325, "rtiHandle in"=w333) -> ("error out"=w334:errorcluster, "objectClassHandle"=w319:u64, "rtiHandle out"=w332:i64)  [unwired: 6 in]
                    n94 = call "build map_object_key.vi"("objectClassHandle"=w319, "instanceId"=w318) -> ("object_map_key"=w321:T7)  [unwired: 9 in]
                    n95 = call <vilib>:"get Attribute Handle.vi"("error in"=w334, "attribute name"=w331, "objectClassHandle in"=w319, "rtiHandle in"=w332) -> ("error out"=w323:errorcluster, "attributeHandle"=w326:u64, "rtiHandle out"=w330:i64)  [unwired: 4 in, 1 out]
                    n96 = in-place {
                      in-place-border: w328 -> [w351]
                      in-place-border: w326 -> [w348]
                      in-place-border: w323 -> [w346]
                      in-place-border: [w344] -> w322
                      in-place-border: w320 -> [w343]
                      in-place-border: w318 -> [w339]
                      in-place-border: w314 -> [w338]
                      in-place-border: w315 -> [w337]
                      in-place-border: w314 -> [w336]
                      n97 = in-place-match #9(w317) -> (w341:T12)
                      n98 = in-place-map #10(w329, w321) -> (w350:T8, w352:bool)  [unwired: 1 in]
                      n99 = case shown="True" w352 {
                        tunnel: w351 -> [_ w369]
                        tunnel: w350 -> [w363 w368]
                        tunnel: [w363 w367] -> w349
                        tunnel: w346 -> [w362 w366]
                        tunnel: [w362 w365] -> w345
                        tunnel: w343 -> [_ w364]
                        frame False {
                        }
                        frame True {
                          n100 = call "Initialize Object Map.vi"("error in"=w366, "vsObjectId"=w364, "status channel map"=w369, "object map in"=w368) -> ("error out"=w365:errorcluster, "object map out"=w367:T8)  [unwired: 6 in]
                        }
                      }
                      n101 = Insert Into Map(map in=w341, key=w338, value=w339) -> (map out=w340:T12)  [unwired: 2 out]
                      n102 = in-place {
                        in-place-border: w348 -> [w357]
                        in-place-border: w345 -> [w361]
                        in-place-border: [w360] -> w344
                        in-place-border: w337 -> [w354]
                        in-place-border: w336 -> [w353]
                        n103 = in-place-cluster #11(w349) -> ("attrHandleSet"=w359:u64, "attributeMap"=w358:map{u64, T5})
                        n104 = call <vilib>:"Insert Element to Attribute Handle Set.vi"("error in"=w361, "attributeHandle"=w357, "attrHandleSet in"=w359) -> ("error out"=w360:errorcluster, "attrHandleSet out"=w355:u64)  [unwired: 6 in, 1 out]
                        n105 = call "Initialize Attribute-Parameter Map.vi"("vs channel index"=w353, "dataType"=w354, "parameterHandle"=w357, "Map in"=w358) -> ("Map out"=w356:map{u64, T5})  [unwired: 7 in]
                        n106 = in-place-cluster #11("attrHandleSet"=w355, "attributeMap"=w356) -> (w347:T8)
                      }
                      n107 = in-place-map #10(w347, LVMapReplaceAction."Add or Modify Entry" ("action")) -> (w327:T6)  [unwired: 2 out]
                      n108 = in-place-match #9(w340) -> (w316:T12)
                    }
                  }
                  n109 = Bundle By Name(cluster=w308, "hlaMap.out_map_vs_ch_instanceId"=w299, "hlaMap.out_objectMap"=w305) -> (w306:T1)
                  n110 = call "LogErrInfo.vi"("location info"="OnOutObjectMap", "error in (no error)"=w304) -> ("error out"=w303:errorcluster)  [unwired: 9 in]
                }
              }
            }
          }
          frame "Object Management" {
            # "Publish objects and interactions"
            # "Subscribe to interactions and objects"
            n111 = Unbundle By Name(w379) -> ("hlaMap.out_objectMap"=w370:T6, "hlaMap.out_interactionMap"=w376:T3, "hlaMap.in_objectMap"=w382:T6, "hlaMap.in_interactionMap"=w388:T3)
            n112 = for {
              shift-right: [w415] -> w384
              shift-left: w389 -> [w418]
              tunnel: w388 -> [w414] mode=indexing
              shift-right: [w416] -> w385
              shift-left: w387 -> [w417]
              n113 = Unbundle By Name(w414) -> ("objectClassHandle"=w413:u64)
              n114 = call <vilib>:"subscribe Interaction Class.vi"("error in"=w418, "active (T)"=TRUE, "ineractionClassHandle in"=w413, "rtiHandle in"=w417) -> ("error out"=w415:errorcluster, "rtiHandle out"=w416:i64)  [unwired: 5 in, 1 out]
            }
            n115 = for {
              shift-right: [w408] -> w377
              shift-left: w384 -> [w411]
              tunnel: w382 -> [w407] mode=indexing
              shift-right: [w409] -> w378
              shift-left: w385 -> [w410]
              n116 = Unbundle By Name(w407) -> ("map_object_key.objectClassHandle"=w406:u64, "attributeMap.attrHandleSet"=w405:u64)
              n117 = call <vilib>:"subscribe Object Class Attributes.vi"("active (T)"=TRUE, "error in"=w411, "attributeHandleSet in"=w405, "objectClassHandle in"=w406, "rtiHandle in"=w410) -> ("error out"=w408:errorcluster, "rtiHandle out"=w409:i64)  [unwired: 3 in, 2 out]
            }
            n118 = for {
              shift-right: [w401] -> w374
              shift-left: w377 -> [w404]
              tunnel: w376 -> [w400] mode=indexing
              shift-right: [w402] -> w373
              shift-left: w378 -> [w403]
              n119 = Unbundle By Name(w400) -> ("objectClassHandle"=w399:u64)
              n120 = call <vilib>:"publish Interaction Class.vi"("error in"=w404, "ineractionClassHandle in"=w399, "rtiHandle in"=w403) -> ("error out"=w401:errorcluster, "rtiHandle out"=w402:i64)  [unwired: 6 in, 1 out]
            }
            n121 = for {
              shift-right: [w395] -> w372
              shift-left: w374 -> [w398]
              tunnel: w370 -> [w394] mode=indexing
              shift-right: [w396] -> w371
              shift-left: w373 -> [w397]
              n122 = Unbundle By Name(w394) -> ("map_object_key.objectClassHandle"=w393:u64, "attributeMap.attrHandleSet"=w392:u64)
              n123 = call <vilib>:"publish Object Class Attributes.vi"("error in"=w398, "attributeHandleSet in"=w392, "objectClassHandle in"=w393, "rtiHandle in"=w397) -> ("error out"=w395:errorcluster, "rtiHandle out"=w396:i64)  [unwired: 4 in, 2 out]
            }
            n124 = call <vilib>:"register Callbacks.vi"("error in"=w372, "rtiHandle in"=w371) -> ("error out"=w383:errorcluster, "federate events"=w380:refnum<event-registration>, "rtiHandle out"=w386:i64)  [unwired: 7 in]
            n125 = Bundle By Name(cluster=w379, "hla event registration"=w380) -> (w381:T1)
          }
          frame "Start" {
            n126 = call <vilib>:"start RTI ambassador.vi"("error in"=w427, "rtiHandle in"=w426) -> ("error out"=w423:errorcluster, "rtiHandle out"=w425:i64)  [unwired: 8 in]
          }
          frame "RegisterObjectInstances" {
            n127 = Unbundle By Name(w432) -> ("hlaMap.out_map_vs_ch_objectInstance"=w438:T13, "hlaMap.out_objectMap"=w442:T6, "rtiHandle"=w444:i64)
            n128 = Generate Occurrence() -> (w434:refnum<k4>)
            n129 = for {
              shift-right: [w465] -> w441
              shift-left: w445 -> [w481]
              tunnel: w444 -> [w480]
              tunnel: w442 -> [w475] mode=indexing
              tunnel: w439 -> [w472]
              shift-right: [w467] -> w436
              shift-left: w438 -> [w468]
              shift-right: [w466] -> w435
              shift-left: w434 -> [w466]
              # "out: instance name, objectclass, intance"
              # "in: instance name, objectclass"
              n130 = Unbundle By Name(w475) -> ("map_object_key.instanceId"=w469:i32, "map_object_key.objectClassHandle"=w474:u64, "attributeMap.objectInstancePrefix"=w473:string)
              n131 = call "build unique object Insance name.vi"("object instance prefix"=w473) -> ("object instance name"=w460:string)  [unwired: 10 in]
              n132 = call <vilib>:"reserve Object Instance Name.vi"("error in"=w481, "theObjectInstanceName"=w460, "rtiHandle in"=w480) -> ("error out"=w463:errorcluster, "rtiHandle out"=w477:i64)  [unwired: 7 in]
              n133 = call "LogErrInfo.vi"("location info"="OnReservingName", "error in (no error)"=w463) -> ("error out"=w462:errorcluster)  [unwired: 9 in]
              n134 = Wait on Notification(notifier=w472, timeout in ms (-1)=10000, error in (no error)=w462) -> (notification=w478:T27, error out=w476:errorcluster)  [unwired: 1 in, 2 out]
              n135 = Unbundle By Name(w478) -> ("objInstanceName"=w479:string, "success"=w470:bool)
              n136 = case shown="True" w470 {
                tunnel: [w484 w485] -> w482
                tunnel: w479 -> [_ w492]
                tunnel: w477 -> [_ w495]
                tunnel: w476 -> [w484 w494]
                tunnel: w474 -> [_ w493]
                tunnel: w469 -> [_ w488]
                tunnel: w468 -> [w483 w489]
                tunnel: [w483 w487] -> w467
                frame False {
                }
                frame True {
                  n137 = call <vilib>:"register Object Instance.vi"("error in"=w494, "objectInstanceName"=w492, "objectClassHandle in"=w493, "rtiHandle in"=w495) -> ("error out"=w486:errorcluster, "objectInstanceHandle"=w490:u64, "objectClassHandle out"=w491:u64)  [unwired: 4 in, 1 out]
                  n138 = case shown="No Error" w486 {
                    selector: w486 -> [w501 w511]
                    tunnel: w492 -> [w496 _]
                    tunnel: w491 -> [w497 _]
                    tunnel: w490 -> [w498 _]
                    tunnel: w489 -> [w504 w510]
                    tunnel: w488 -> [w503 _]
                    tunnel: [w502 w510] -> w487
                    tunnel: [w501 w511] -> w485
                    frame No Error {
                      n139 = disable-structure shown="Enabled" {
                        disable-tunnel: w498 -> [w507 _]
                        disable-tunnel: w497 -> [w506 _]
                        disable-tunnel: w496 -> [w505 _]
                        frame Enabled {
                          n140 = Format Into String(format string="object inst %d h %d registered: %s", w507, w506, w505) -> (resulting string=w508:string)  [unwired: 2 in, 1 out]
                          n141 = call "LogToSyslog.vi"("message"=w508) -> ()  [unwired: 9 in, 2 out]
                        }
                        frame Disabled {
                        }
                      }
                      n142 = Bundle By Name(cluster=T14 {"objectInstanceHandle"=0, "objectClassHandle"=0} ("value"), "objectInstanceHandle"=w498, "objectClassHandle"=w497) -> (w499:T14)
                      n143 = Insert Into Map(map in=w504, key=w503, value=w499) -> (map out=w502:T13)  [unwired: 2 out]
                    }
                    frame Error {
                    }
                  }
                }
              }
              n144 = call "LogErrInfo.vi"("location info"="OnRegisteringObjectInstance", "error in (no error)"=w482) -> ("error out"=w465:errorcluster)  [unwired: 9 in]
            }
            n145 = while {
              tunnel: w443 -> [w519]
              tunnel: [w518] -> w446
              tunnel: w445 -> [_]
              tunnel: w439 -> [w516]
              tunnel: w434 -> [w514]
              shift-right: [w512] -> w429
              shift-left: T29[] [] ("Array") -> [w513]
              stop <- w517 stop-if-true
              n146 = event shown="[2] <discoverObjectInstance>: User Event" {
                selector: w519 -> [_ _ _ _ _]
                dyn-events: [_ _ _ _ _] -> w518
                timeout: 200 -> [_ _ _ _ _]
                tunnel: [w521 _ _ _ _] -> w517
                tunnel: w516 -> [_ w528 _ _ w555]
                tunnel: w514 -> [w525 _ _ _ _]
                tunnel: w513 -> [w520 w526 w539 w549 w550]
                tunnel: [w520 w526 w538 w547 w550] -> w512
                event Timeout {
                  n147 = event-data() -> ()  [unwired: 1 in, 1 out]
                  n148 = Wait on Occurrence(1:FALSE ("ignore previous (T)"), 2:w525, 3:0 ("ms timeout (-1)")) -> (0:w522:bool)
                  n149 = Not(x=w522) -> (.not. x?=w521:bool)
                }
                event User Event {
                  n150 = event-data() -> ("objInstNameResSucc"=w527:string)  [unwired: 1 in]
                  n151 = Bundle By Name(cluster=T27 {"objInstanceName"="", "success"=FALSE} ("notification"), "objInstanceName"=w527, "success"=TRUE) -> (w530:T27)
                  n152 = Send Notification(notification=w530, notifier=w528) -> ()  [unwired: 1 in, 2 out]
                  n153 = disable-structure shown="DEBUG==True" {
                    disable-tunnel: w527 -> [_ w532]
                    frame condition #0 {
                    }
                    frame condition #1 (active) {
                      n154 = Format Into String(format string="Successfully registered %s name", w532) -> (resulting string=w533:string)  [unwired: 2 in, 1 out]
                      n155 = call "LogToSyslog.vi"("message"=w533) -> ()  [unwired: 9 in, 2 out]
                    }
                  }
                }
                event User Event {
                  n156 = event-data() -> ("objectClassHandle"=w536:u64, "objectInstanceHandle"=w535:u64, "objectInstanceName"=w541:T30, "size"=w540:u32)  [unwired: 1 in, 1 out]
                  n157 = call <vilib>:"objectInstance Cluster to String.vi"("size"=w540, "string cluster in"=w541) -> ("string out"=w537:string)  [unwired: 9 in]
                  n158 = disable-structure shown="Enabled" {
                    disable-tunnel: w535 -> [w544 _]
                    disable-tunnel: w536 -> [w543 _]
                    disable-tunnel: w537 -> [w542 _]
                    frame Enabled {
                      n159 = Format Into String(format string="object inst %d h %d discovered (init): %s", w544, w543, w542) -> (resulting string=w545:string)  [unwired: 2 in, 1 out]
                      n160 = call "LogToSyslog.vi"("message"=w545) -> ()  [unwired: 9 in, 2 out]
                    }
                    frame Disabled {
                    }
                  }
                  n161 = call "Add incoming ObjectInstance Record.vi"("objectClassHandle"=w536, "objectInstanceHandle"=w535, "objectInstanceName"=w537, "object instance records in"=w539) -> ("object instance records out"=w538:T29[])  [unwired: 7 in]
                }
                event User Event {
                  n162 = event-data() -> ("objectInstanceHandle"=w548:u64)  [unwired: 1 in]
                  n163 = call "Delete incoming ObjectInstance Record.vi"("objectInstanceHandle"=w548, "Array in"=w549) -> ("Array out"=w547:T29[])  [unwired: 8 in, 1 out]
                }
                event User Event {
                  n164 = event-data() -> ("objInstNameResFail"=w551:string)  [unwired: 1 in]
                  n165 = Bundle By Name(cluster=T27 {"objInstanceName"="", "success"=FALSE} ("notification"), "objInstanceName"=w551, "success"=FALSE) -> (w553:T27)
                  n166 = Send Notification(notification=w553, notifier=w555) -> ()  [unwired: 1 in, 2 out]
                  n167 = disable-structure shown="DEBUG==True" {
                    disable-tunnel: w551 -> [_ w556]
                    frame condition #0 {
                    }
                    frame condition #1 (active) {
                      n168 = Format Into String(format string="Failed to Register%s name", w556) -> (resulting string=w557:string)  [unwired: 2 in, 1 out]
                      n169 = call "LogToSyslog.vi"("message"=w557) -> ()  [unwired: 9 in, 2 out]
                    }
                  }
                }
              }
            }
            n170 = Array Size(array=w429) -> (size(s)=w430:i32)
            n171 = case shown="Default" w430 {
              tunnel: w432 -> [w450 w453]
              tunnel: [w450 w452] -> w431
              tunnel: w429 -> [_ w451]
              frame 0 {
              }
              frame Default {
                n172 = in-place {
                  in-place-border: w451 -> [w454]
                  n173 = in-place-cluster #12(w453) -> ("hlaMap"=w456:T2)
                  n174 = for {
                    shift-right: [w458] -> w455
                    shift-left: w456 -> [w459]
                    tunnel: w454 -> [w457] mode=indexing
                    n175 = call "Add Discovered Object Instance (incoming).vi"("discoverObjInstance"=w457, "hlaMap in"=w459) -> ("hlaMap out"=w458:T2)  [unwired: 9 in]
                  }
                  n176 = in-place-cluster #12("hlaMap"=w455) -> (w452:T1)
                }
              }
            }
            n177 = Set Occurrence(w435) -> ()
            n178 = Bundle By Name(cluster=w431, "hlaMap.out_map_vs_ch_objectInstance"=w436) -> (w437:T1)
            n179 = Release Notifier(notifier=w439, error in (no error)=w441) -> (error out=w440:errorcluster)  [unwired: 1 in, 2 out]
          }
        }
        n180 = Or(x=w19, y=w20) -> (x .or. y?=w18:bool)
      }
    }
    frame Error {
    }
  }
  "error out" <- w2
  "inline runtime data" <- w1
  "Device Reference out" <- "Device Reference in"
  "settings out" <- "settings in"
